vi "Teardown.vi"(8 "Error In":errorcluster, 11 "Listener":refnum<class "Listener.lvclass">) -> (0 "Error Out":errorcluster)   [LabVIEW 2018, in "Tests.lvlib" / "Listener.lvlib"]
uses:
  Listener.lvlib
  src/Toolkit/Listener/Listener.lvclass
  src/Toolkit/Listener/Support/Destroy to Session.vi
  src/Toolkit/Session/Session.lvclass
  src/Toolkit/SSH/SSH.lvclass
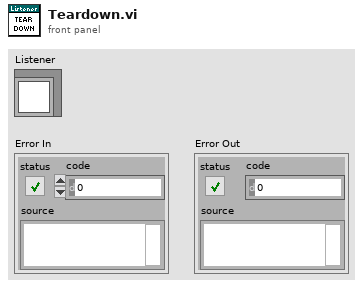
[diagram p1: front panel]
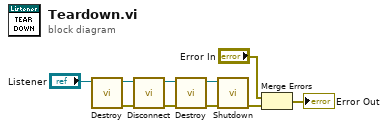
[diagram p0: block diagram]
diagram:
  n1 = call-poly "Destroy.vi"("Listener"="Listener") -> ("Error Out"=w1:errorcluster, "Session"=w2:refnum<class "Session.lvclass">)  [unwired: 9 in]
  n2 = call "Disconnect.vi"("Error In"=w1, "Session In"=w2) -> ("Error Out"=w10:errorcluster, "Sesssion Out"=w9:refnum<class "Session.lvclass">)  [unwired: 8 in]
  n3 = call "Destroy.vi"("Error In"=w10, "Session"=w9) -> ("Error Out"=w7:errorcluster, "SSH"=w6:refnum<class "SSH.lvclass">)  [unwired: 8 in]
  n4 = call "Shutdown.vi"("Error In"=w7, "SSH"=w6) -> ("Error Out"=w8:errorcluster)  [unwired: 9 in]
  n5 = Merge Errors("Error In", w8) -> (→"Error Out":errorcluster)
